vi "Generic VI.vi"(8 "error in (no error)":errorcluster, 11 "VI Reference in":variant) -> (0 "error out":errorcluster, 2 "Generic VI Reference":refnum<vi>, 3 "VI Reference out":variant)   [LabVIEW 2021, in "Thread.lvlib"]
uses:
  Thread.lvlib
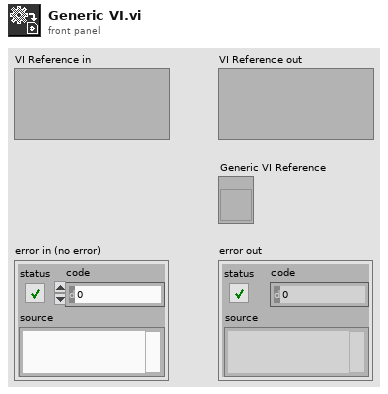
[diagram p1: front panel]
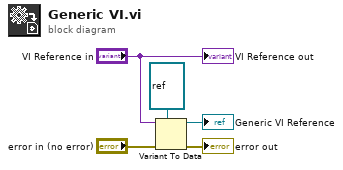
[diagram p0: block diagram]
diagram:
  n1 = Variant To Data(error in="error in (no error)", type=refnum<vi> refnum ("Generic VI Reference"), Variant="VI Reference in") -> (data=→"Generic VI Reference":refnum<vi>, error out=→"error out":errorcluster)
  "VI Reference out" <- "VI Reference in"
